vi "Solenoid - DRAIN.vi"(6 "Debug":bool, 8 "Error In":errorcluster, 9 "HEWH MW100 Channel Numbers":T2="011", 10 "Drain/Purge Valve":T1, 11 "VISA session":refnum<visa-resource-name>="MW100") -> (0 "Error Out":errorcluster, 3 "dup VISA session":refnum<visa-resource-name>)   [LabVIEW 2023]
uses:
  Type Definitions/HEWH MW100 Channel Numbers.ctl
  Type Definitions/HEWH Normally Closed Valve Control.ctl
panel:
  out "Message":string
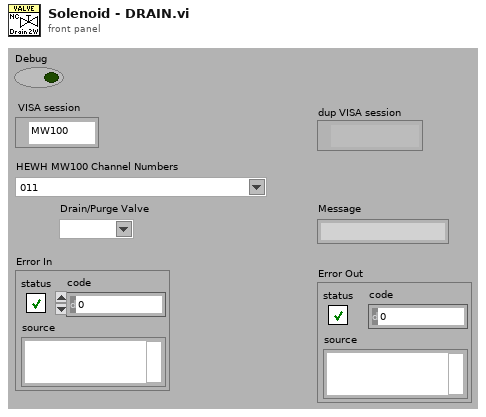
[diagram p1: front panel]
types:
  T1 = typedef "HEWH Normally Closed Valve Control.ctl" = string
  T2 = typedef "HEWH MW100 Channel Numbers.ctl" = string
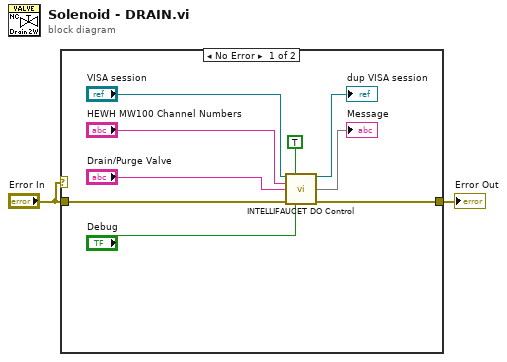
[diagram p0: block diagram]
diagram:
  n1 = case shown="No Error" "Error In" {
    tunnel: "Error In" -> [w8 w12]
    tunnel: [w9 w12] -> w2
    frame No Error {
      n2 = call "INTELLIFAUCET DO Control.vi"("VISA session"="VISA session", 1:TRUE ("Normally Closed Valve?"), "HEWH MW100 Channel Numbers"="HEWH MW100 Channel Numbers", "Normally Open"="Drain/Purge Valve", "Error In"=w8, 12:"Debug") -> ("dup VISA session"=→"dup VISA session":refnum<visa-resource-name>, 8:→"Message", "error out"=w9:errorcluster)  [unwired: 7 in]
    }
    frame Error {
    }
  }
  "Error Out" <- w2
